vi "CTRE_PigeonIMU_GetAccelerometerAngles.vi"(8 "error in (no error)":errorcluster, 11 "PigeonIMUDevRef":T2={"DeviceStatus"={"status"=FALSE, "code"=0, "source"=""}, "Device Number"=0, "Type"=352321536, "Device ID"=0, "Handle"=0, "UsageFrame"=0, "Library Path"=path ""} {"Type" items=["CAN"=352321536, "TalonSRX"=33554432]}) -> (0 "error out":errorcluster, 2 "Accelerometer Angles":T1, 3 "PigeonIMUDevRef":T2={"DeviceStatus"={"status"=FALSE, "code"=0, "source"=""}, "Device Number"=0, "Type"=352321536, "Device ID"=0, "Handle"=0, "UsageFrame"=0, "Library Path"=path ""} {"Type" items=["CAN"=352321536, "TalonSRX"=33554432]})   [LabVIEW 2016]
uses:
  <vilib>/Rock Robotics/WPI/ThirdParty/Sensors/Pigeon IMU/CTRE_PigeonIMU_DeviceRef.ctl
  <vilib>/Rock Robotics/WPI/ThirdParty/Sensors/Pigeon IMU/CTRE_PigeonIMU_ConnectionType.ctl
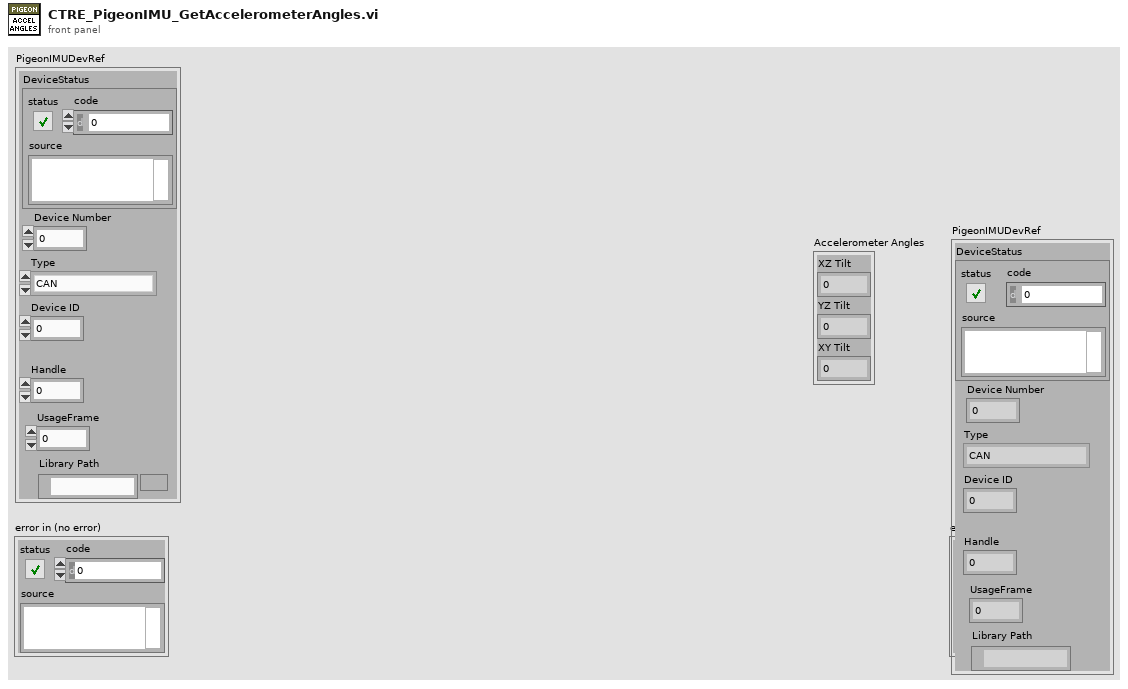
[diagram p1: front panel]
types:
  T1 = cluster{"XZ Tilt":dbl, "YZ Tilt":dbl, "XY Tilt":dbl}
  T2 = typedef "CTRE_PigeonIMU_DeviceRef.ctl" = cluster{"DeviceStatus":errorcluster, "Device Number":u8, "Type":T3, "Device ID":u32, "Handle":u64, "UsageFrame":u32, "Library Path":path}
  T3 = typedef "CTRE_PigeonIMU_ConnectionType.ctl" = u32
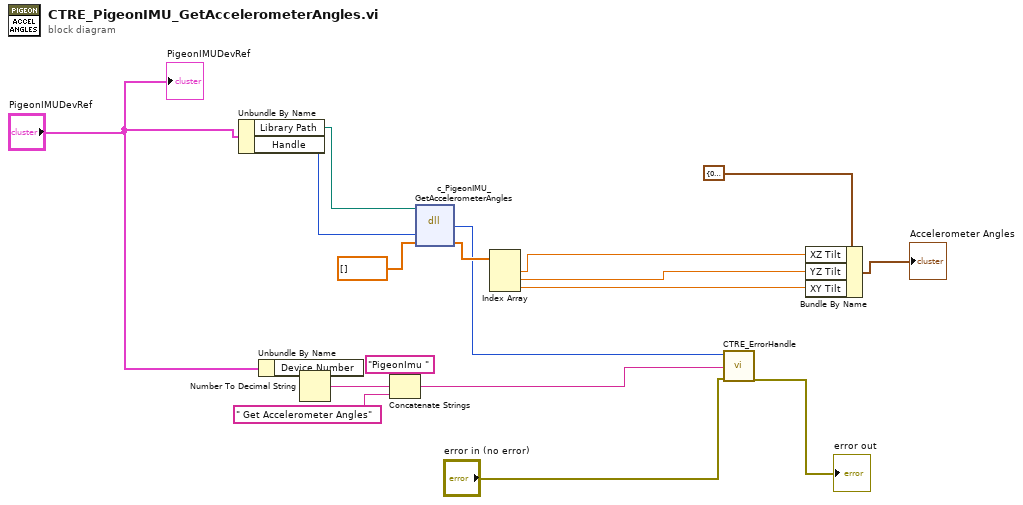
[diagram p0: block diagram]
diagram:
  n1 = Unbundle By Name("PigeonIMUDevRef") -> ("Library Path"=w17:path, "Handle"=w18:u64)
  n2 = Unbundle By Name("PigeonIMUDevRef") -> ("Device Number"=w9:u8)
  n3 = Number To Decimal String(number=w9) -> (decimal integer string=w8:string)  [unwired: 1 in]
  n4 = Concatenate Strings("PigeonImu " ("string"), w8, " Get Accelerometer Angles" ("string")) -> (w2:string)
  n5 = dll-call lib="?" fn="c_PigeonIMU_GetAccelerometerAngles"(path in=w17, "handle"=w18, "tiltAngles"=dbl[] []) -> ("return type"=w1:i32, "tiltAngles"=w13:dbl[])  [unwired: 3 in, 2 out]
  n6 = Index Array(array=w13) -> (element #1=w12:dbl, element #2=w11:dbl, element #3=w10:dbl)  [unwired: 3 in]
  n7 = call <vilib>:"CTRE_ErrorHandle.vi"("error in"="error in (no error)", "origin"=w2, "code"=w1) -> ("error out"=→"error out":errorcluster)  [unwired: 8 in]
  n8 = Bundle By Name(cluster=T1 {"XZ Tilt"=0.0, "YZ Tilt"=0.0, "XY Tilt"=0.0} ("Angles"), "XZ Tilt"=w12, "YZ Tilt"=w11, "XY Tilt"=w10) -> (→"Accelerometer Angles":T1)
  "PigeonIMUDevRef" <- "PigeonIMUDevRef"
